vi "SolveMurphKoop.vi"(6 "P":dbl=1013.25, 8 "Error In":errorcluster, 9 "Type":enum16{"Ice", "Water"}(ring)=enum."Water", 10 "T":dbl, 11 "RH":dbl=100.0) -> (0 "Error Out":errorcluster, 1 "wv":dbl, 2 "es":dbl, 3 "e":dbl)   [LabVIEW 2014, in "Atmospheric Library.lvlib"]
doc: "Solves the equations in Murphy and Koop [2005] for 1) the saturation vapor pressure over ice/water, 2) the water vapor partial pressure (based on the input <B>RH</B>) and the water vapor mixing ratio (based on <B>P</B> and <B>RH</B>). If no pressure is given, then wv will return NaN. If the <B>T</B> > 0 degrees Celsius, and the <B>Type</B> of calculation is for ice, then this function will throw an error."
uses:
  Atmospheric Library.lvlib
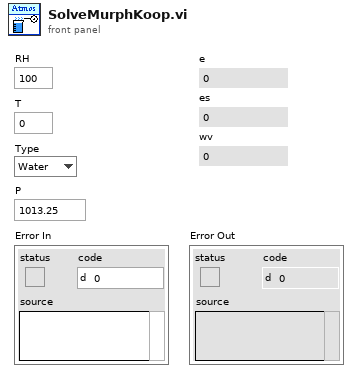
[diagram p1: front panel]
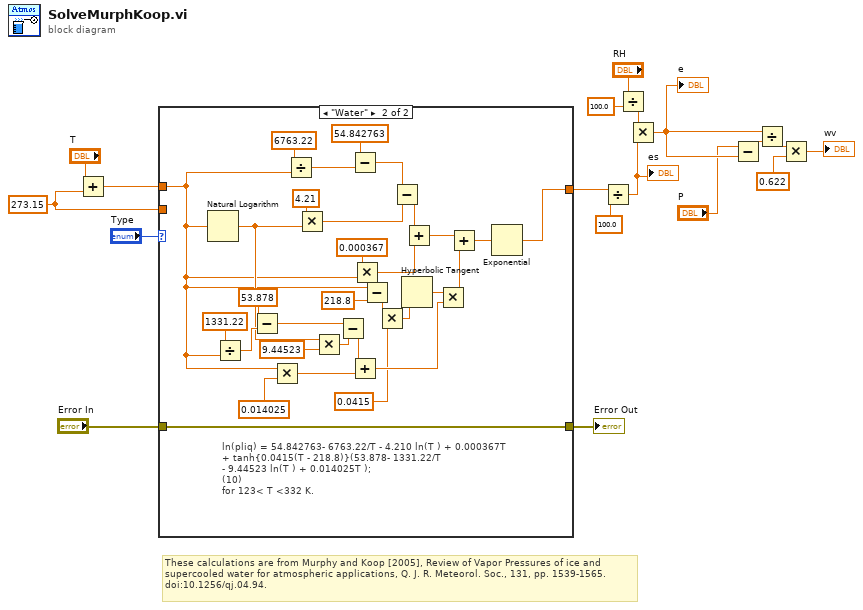
[diagram p0: block diagram]
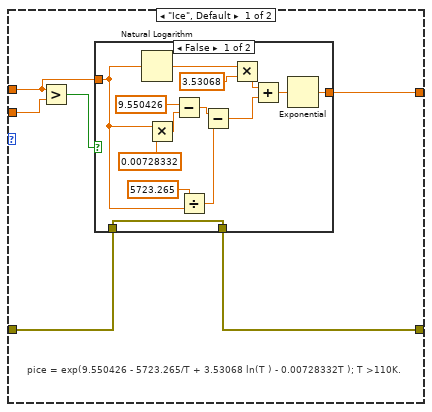
[diagram p2: hidden frame]
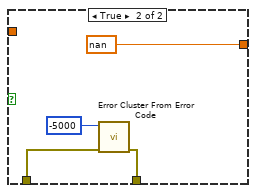
[diagram p3: hidden frame]
diagram:
  w16 = 273.15
  # "These calculations are from Murphy and Koop [2005], Review of Vapor Pressures of ice and supercooled water for atmospheric applications, Q. J. R. Meteorol. Soc., 131, pp. 1539-1565. doi:10.1256/qj.04.94."
  n1 = Add(x="T", y=w16) -> (x+y=w15:dbl)
  n2 = case shown="\"Water\"" "Type" {
    tunnel: w16 -> [w23 _]
    tunnel: w15 -> [w22 w53]
    tunnel: [w21 w50] -> w9
    tunnel: "Error In" -> [w20 w46]
    tunnel: [w19 w46] -> w10
    frame "Ice", Default {
      # "pice = exp(9.550426 - 5723.265/T + 3.53068 ln(T ) - 0.00728332T ); T >110K."
      n3 = Greater?(x=w22, y=w23) -> (0:w24:bool)
      n4 = case shown="False" w24 {
        tunnel: w22 -> [w37 _]
        tunnel: [w27 nan] -> w21
        tunnel: w20 -> [w25 w41]
        tunnel: [w25 w39] -> w19
        frame False {
          n5 = Natural Logarithm(1:w37) -> (0:w35:dbl)
          n6 = Multiply(x=w37, y=0.00728332) -> (x*y=w31:dbl)
          n7 = Subtract(x=9.550426, y=w31) -> (x-y=w30:dbl)
          n8 = Divide(x=5723.265, y=w37) -> (x/y=w29:dbl)
          n9 = Subtract(x=w30, y=w29) -> (x-y=w28:dbl)
          n10 = Multiply(x=w35, y=3.53068) -> (x*y=w33:dbl)
          n11 = Add(x=w33, y=w28) -> (x+y=w26:dbl)
          n12 = Exponential(1:w26) -> (0:w27:dbl)
        }
        frame True {
          n13 = call <vilib>:"Error Cluster From Error Code.vi"("error in (no error)"=w41, "error code (0)"=-5000) -> ("error out"=w39:errorcluster)  [unwired: 7 in]
        }
      }
    }
    frame "Water" {
      # "ln(pliq) = 54.842763- 6763.22/T - 4.210 ln(T ) + 0.000367T\n+ tanh{0.0415(T - 218.8)}(53.878- 1331.22/T\n- 9.44523 ln(T ) + 0.014025T );\n(10)\nfor 123< T <332 K."
      n14 = Natural Logarithm(1:w53) -> (0:w58:dbl)
      n15 = Divide(x=1331.22, y=w53) -> (x/y=w62:dbl)
      n16 = Subtract(x=53.878, y=w62) -> (x-y=w55:dbl)
      n17 = Multiply(x=w53, y=0.014025) -> (x*y=w54:dbl)
      n18 = Divide(x=6763.22, y=w53) -> (x/y=w69:dbl)
      n19 = Multiply(x=4.21, y=w58) -> (x*y=w67:dbl)
      n20 = Multiply(x=w58, y=9.44523) -> (x*y=w56:dbl)
      n21 = Subtract(x=w55, y=w56) -> (x-y=w57:dbl)
      n22 = Subtract(x=54.842763, y=w69) -> (x-y=w68:dbl)
      n23 = Add(x=w57, y=w54) -> (x+y=w51:dbl)
      n24 = Multiply(x=0.000367, y=w53) -> (x*y=w65:dbl)
      n25 = Subtract(x=w53, y=218.8) -> (x-y=w44:dbl)
      n26 = Multiply(x=w44, y=0.0415) -> (x*y=w43:dbl)
      n27 = Subtract(x=w68, y=w67) -> (x-y=w66:dbl)
      n28 = Hyperbolic Tangent(1:w43) -> (0:w63:dbl)
      n29 = Add(x=w66, y=w65) -> (x+y=w49:dbl)
      n30 = Multiply(x=w63, y=w51) -> (x*y=w48:dbl)
      n31 = Add(x=w49, y=w48) -> (x+y=w47:dbl)
      n32 = Exponential(1:w47) -> (0:w50:dbl)
    }
  }
  "Error Out" <- w10
  n33 = Divide(x=w9, y=100.0) -> (x/y=w7:dbl)
  "es" <- w7
  n34 = Divide(x="RH", y=100.0) -> (x/y=w12:dbl)
  n35 = Multiply(x=w12, y=w7) -> (x*y=w2:dbl)
  "e" <- w2
  n36 = Subtract(x="P", y=w2) -> (x-y=w6:dbl)
  n37 = Divide(x=w2, y=w6) -> (x/y=w5:dbl)
  n38 = Multiply(x=w5, y=0.622) -> (x*y=→"wv":dbl)
